vi "random_source.vi"(4 "error in (no error)":errorcluster, 7 "Modulation Parameters In":T1 {"TX Parameters"."TX Sample Rate" items=["4M"]}) -> (0 "error out":errorcluster, 2 "output bit stream":u8[](array[numeric]), 3 "Modulation Parameters Out":T1 {"TX Parameters"."TX Sample Rate" items=["4M"]})   [LabVIEW 2012]
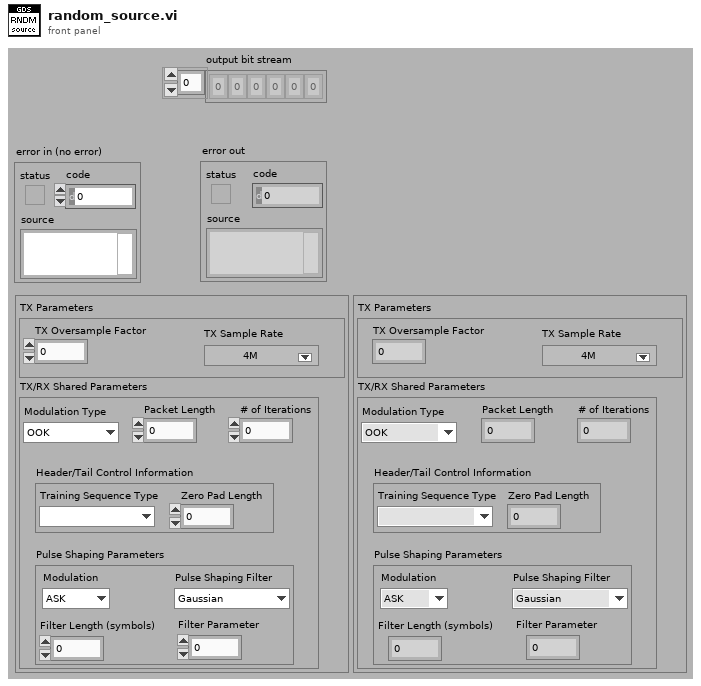
[diagram p1: front panel]
types:
  T1 = cluster{"TX Parameters":cluster{"TX Oversample Factor":u16, "TX Sample Rate":dbl}, "TX/RX Shared Parameters":cluster{"Modulation Type":enum16{"OOK", "FSK"}, "Packet Length":u32, "# of Iterations":dbl, "Pulse Shaping Parameters":cluster{"Modulation":enum16{"ASK", "FSK", "PSK", "QAM", "MSK", "PAM"}, "Pulse Shaping Filter":enum16{"Gaussian"}, "Filter Length (symbols)":dbl, "Filter Parameter":dbl}, "Header/Tail Control Information":cluster{"Training Sequence Type":enum16{""}, "Zero Pad Length":dbl}}}
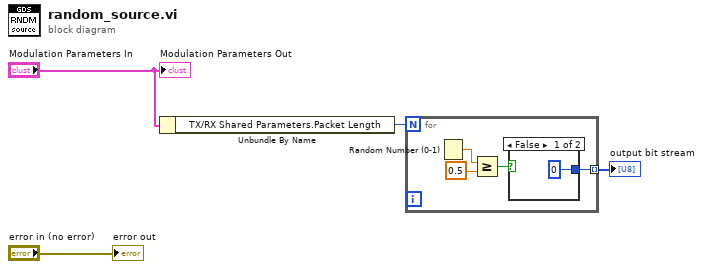
[diagram p0: block diagram]
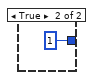
[diagram p2: hidden frame]
diagram:
  n1 = Unbundle By Name("Modulation Parameters In") -> ("TX/RX Shared Parameters.Packet Length"=w1:u32)
  n2 = for {
    N: w1 -> [_]
    tunnel: [w5] -> w4 mode=indexing
    n3 = Random Number (0-1)() -> (number: 0 to 1=w7:dbl)
    n4 = Greater Or Equal?(x=w7, y=0.5) -> (x >= y?=w6:bool)
    n5 = case shown="False" w6 {
      tunnel: [u8 0 u8 1] -> w5
      frame False {
      }
      frame True {
      }
    }
  }
  "output bit stream" <- w4
  "error out" <- "error in (no error)"
  "Modulation Parameters Out" <- "Modulation Parameters In"
